vi "Format Message.vi"(7 "formatted string":refnum<vi>, 8 "error in":errorcluster, 10 "String Input":string) -> (0 "error out":errorcluster, 2 "Updated Message":string)   [LabVIEW 2021, in "Pop-Up.lvlib" / "Popup.lvclass"]
doc: "This VI applies special formatting to message strings. The tags are listed below and their purpose:\n\n < b> bold < /b> - without spaces; used so tags will show in context help\n <i> italic </i>\n <strong> bold - strong </strong>\n <em> italic - emphasis </em>\n <del> strikethrough </del>\n <ins> underline </ins>\n <font rgb(#,#,#)> RGB-based color of text </font>"
uses:
  Popup.lvclass
  <vilib>/regexp/Match Regular Expression.xnode
  Popup.lvclass/Popup.ctl
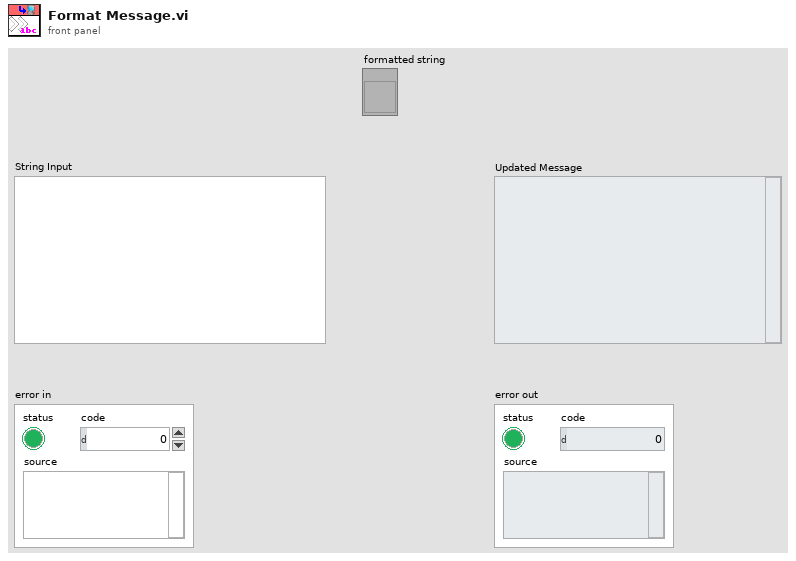
[diagram p1: front panel]
types:
  T1 = cluster{"style":string, "text.selstart":i32, "text.selend":i32}
  T2 = cluster{"style":string, "text.selstart":i32, "text.selend":i32}[]
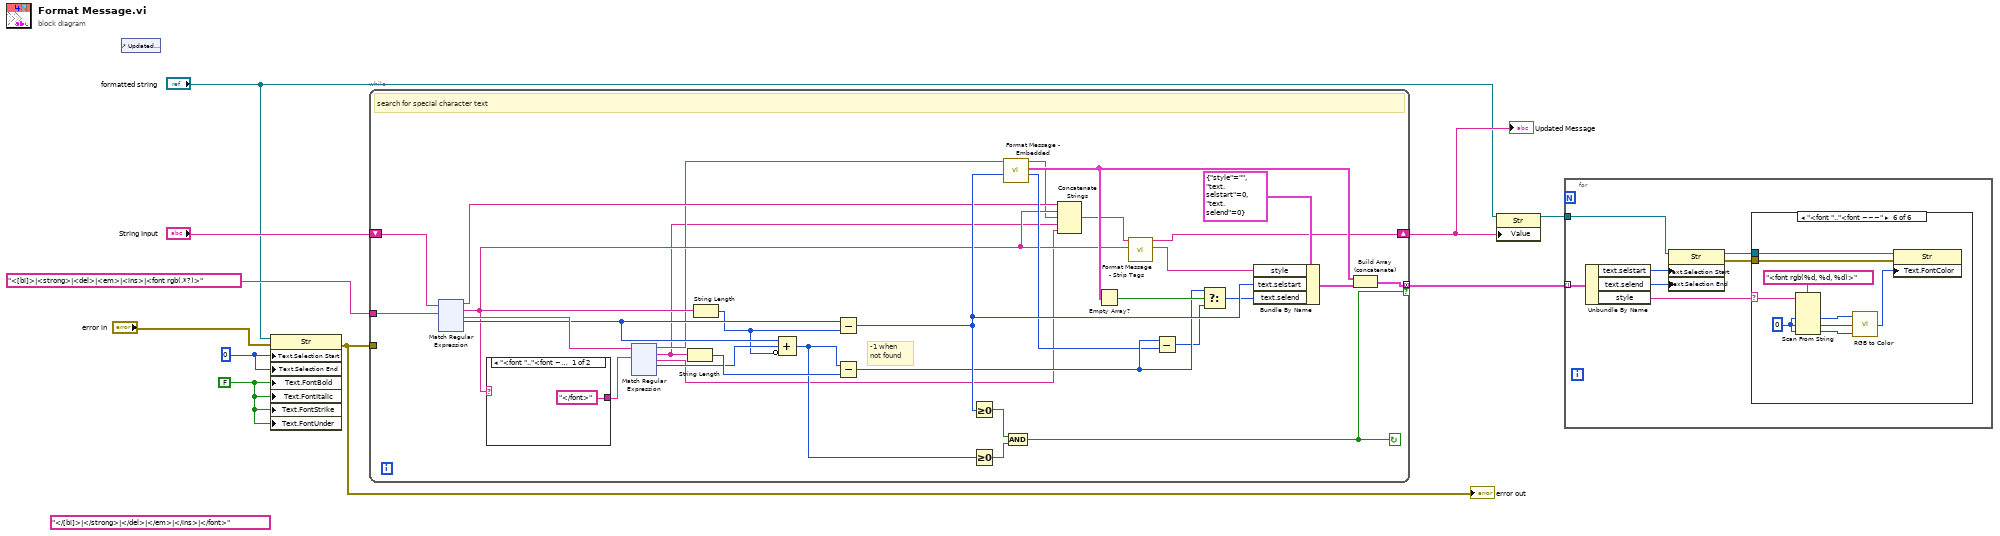
[diagram p0: block diagram]
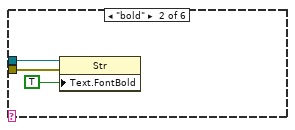
[diagram p3: hidden frame]
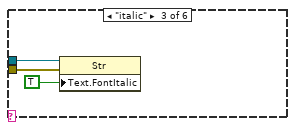
[diagram p4: hidden frame]
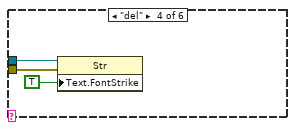
[diagram p5: hidden frame]
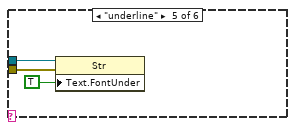
[diagram p6: hidden frame]
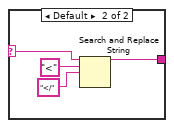
[diagram p7: hidden frame]
diagram:
  (unwired) "</[bi]>|</strong>|</del>|</em>|</ins>|</font>" ("regular expression")
  w8 = u32 0 ("Text.Selection:Start")
  w2 = FALSE ("Text.Font:Bold")
  n1 = control-ref of="Updated Message"() -> ()  [unwired: 1 out]
  n2 = property on="Property Node" class="Str"(reference="formatted string", error in="error in", "Text.Selection Start"=w8, "Text.Selection End"=w8, "Text.FontBold"=w2, "Text.FontItalic"=w2, "Text.FontStrike"=w2, "Text.FontUnder"=w2) -> (error out=w3:errorcluster)  [unwired: 1 out]
  "error out" <- w3
  n3 = while {
    shift-right: [w22] -> w6
    shift-left: "String Input" -> [w25]
    tunnel: [w33] -> w9 mode=concatenating if=w39
    tunnel: w3 -> [_]
    tunnel: "<[bi]>|<strong>|<del>|<em>|<ins>|<font rgb(.*?)>" ("regular expression") -> [w36]
    stop <- w39 continue-if-true
    # "-1 when\nnot found"
    # "search for special character text"
    n4 = xnode "Match Regular Expression"("input string"=w25, "regular expression"=w36) -> ("before match"=w17:string, "whole match"=w16:string, "after match"=w24:string, "offset past match"=w19:i32)  [unwired: 4 in, 1 out]
    n5 = case shown="\"<font \"..\"<font ~~~\"" w16 {
      selector: w16 -> [_ w44]
      tunnel: ["</font>" ("result string") w43] -> w35
      frame "<font ".."<font ~~~" {
      }
      frame Default {
        n6 = Search and Replace String(input string=w44, search string="<", replace string="</" ("replace string (\"\")")) -> (result string=w43:string)  [unwired: 5 in, 3 out]
      }
    }
    n7 = xnode "Match Regular Expression"("input string"=w24, "regular expression"=w35) -> ("before match"=w15:string, "whole match"=w11:string, "after match"=w12:string, "offset past match"=w20:i32)  [unwired: 4 in, 1 out]
    n8 = String Length(string=w11) -> (length=w26:i32)
    n9 = String Length(string=w16) -> (length=w13:i32)
    n10 = Compound Arithmetic op=ADD(w19, w20, invert w13) -> (w18:i32)
    n11 = Subtract(x=w19, y=w13) -> (x-y=w34:i32)
    n12 = Subtract(x=w18, y=w26) -> (x-y=w29:i32)
    n13 = Greater Or Equal To 0?(x=w34) -> (x >= 0?=w40:bool)
    n14 = Greater Or Equal To 0?(x=w18) -> (x >= 0?=w41:bool)
    n15 = call "Format Message - Embedded.vi"("open tag"=w34, "after open tag"=w15) -> ("stripped characters"=w28:i32, "Format Tags"=w31:T2, "stripped string"=w14:string)  [unwired: 7 in]
    n16 = And(x=w40, y=w41) -> (x .and. y?=w39:bool)
    n17 = Concatenate Strings(w17, w16, w14, w11, w12) -> (w23:string)
    n18 = Empty Array?(array=w31) -> (empty?=w32:bool)
    n19 = call "Format Message - Strip Tags.vi"("opening tag"=w16, "after open tag"=w23) -> ("format type"=w21:string, "result string"=w22:string)  [unwired: 8 in]
    n20 = Subtract(x=w29, y=w28) -> (x-y=w27:i32)
    n21 = Select(t=w29, s=w32, f=w27) -> (s? t:f=w30:i32)
    n22 = Bundle By Name(cluster=T1 {"style"="", "text.selstart"=0, "text.selend"=0}, "style"=w21, "text.selstart"=w34, "text.selend"=w30) -> (w37:T1)
    n23 = Build Array (concatenate)(w31, w37) -> (w33:T2)
  }
  "Updated Message" <- w6
  n24 = property class="Str"(reference="formatted string", "Value"=w6) -> (reference out=w5:refnum<vi>)  [unwired: 1 in, 1 out]
  n25 = for {
    tunnel: w9 -> [w287] mode=indexing
    tunnel: w5 -> [w282]
    n26 = Unbundle By Name(w287) -> ("text.selstart"=w286:i32, "text.selend"=w285:i32, "style"=w283:string)
    n27 = property on="Property Node" class="Str"(reference=w282, "Text.Selection Start"=w286, "Text.Selection End"=w285) -> (reference out=w281:refnum<vi>, error out=w284:errorcluster)  [unwired: 1 in]
    n28 = case shown="\"<font \"..\"<font ~~~\"" w283 {
      selector: w283 -> [_ _ _ _ _ w307]
      tunnel: w284 -> [_ w290 w293 w296 w299 w305]
      tunnel: w281 -> [_ w288 w291 w294 w297 w300]
      frame Default {
      }
      frame "bold" {
        n29 = property on="Property Node" class="Str"(reference=w288, error in=w290, "Text.FontBold"=TRUE ("Text.Font:Bold")) -> ()  [unwired: 2 out]
      }
      frame "italic" {
        n30 = property on="Property Node" class="Str"(reference=w291, error in=w293, "Text.FontItalic"=TRUE ("Text.Font:Bold")) -> ()  [unwired: 2 out]
      }
      frame "del" {
        n31 = property on="Property Node" class="Str"(reference=w294, error in=w296, "Text.FontStrike"=TRUE ("Text.Font:Bold")) -> ()  [unwired: 2 out]
      }
      frame "underline" {
        n32 = property on="Property Node" class="Str"(reference=w297, error in=w299, "Text.FontUnder"=TRUE ("Text.Font:Bold")) -> ()  [unwired: 2 out]
      }
      frame "<font ".."<font ~~~" {
        w306 = u8 0 ("default value 2")
        n33 = Scan From String(format string="<font rgb(%d, %d, %d)>", input string=w307, default 1=w306, default 2=w306, default 3=w306) -> (output 1=w303:u8, output 2=w302:u8, output 3=w301:u8)  [unwired: 2 in, 3 out]
        n34 = call <vilib>:"RGB to Color.vi"("B"=w301, "G"=w302, "R"=w303) -> ("Color"=w304:u32)
        n35 = property on="Property Node" class="Str"(reference=w300, error in=w305, "Text.FontColor"=w304) -> ()  [unwired: 2 out]
      }
    }
  }
